vi "get motor settings.vi"(8 "error in (no error)":errorcluster, 10 "motor_settings":T1, 11 "id":i32) -> (0 "error out":errorcluster, 2 "motor_settings out":T1, 3 "function return":i32)   [LabVIEW 2012, in "libximc.lvlib"]
doc: "result_t XIMC_API get_motor_settings (device_t id, motor_settings_t* motor_settings);"
uses:
  libximc.lvlib
  libximc.dll
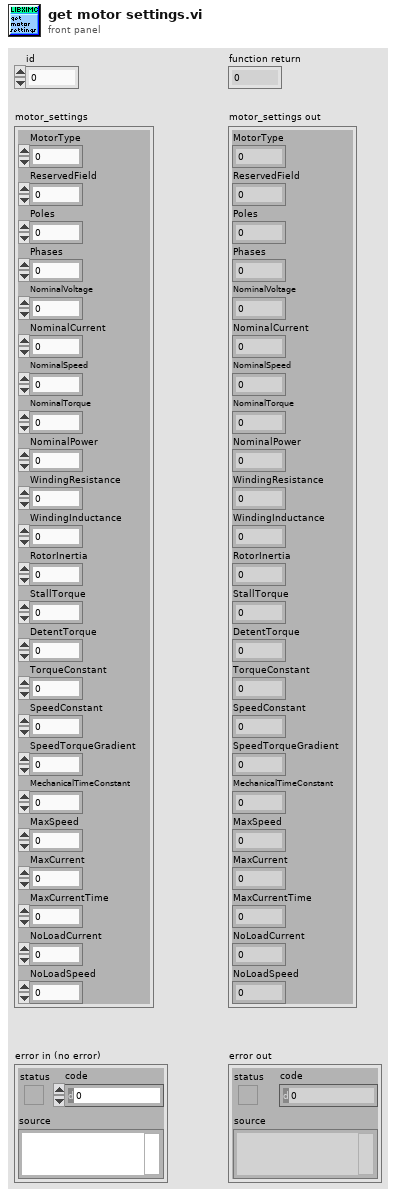
[diagram p1: front panel]
types:
  T1 = cluster{"MotorType":u32, "ReservedField":u32, "Poles":u32, "Phases":u32, "NominalVoltage":sgl, "NominalCurrent":sgl, "NominalSpeed":sgl, "NominalTorque":sgl, "NominalPower":sgl, "WindingResistance":sgl, "WindingInductance":sgl, "RotorInertia":sgl, "StallTorque":sgl, "DetentTorque":sgl, "TorqueConstant":sgl, "SpeedConstant":sgl, "SpeedTorqueGradient":sgl, "MechanicalTimeConstant":sgl, "MaxSpeed":sgl, "MaxCurrent":sgl, "MaxCurrentTime":sgl, "NoLoadCurrent":sgl, "NoLoadSpeed":sgl}
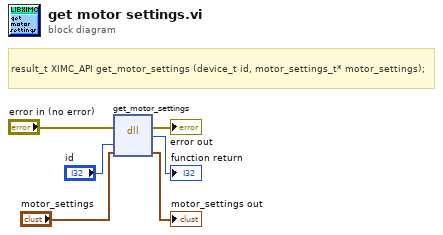
[diagram p0: block diagram]
diagram:
  # "result_t XIMC_API get_motor_settings (device_t id, motor_settings_t* motor_settings);"
  n1 = dll-call lib="E:/labview-2.12.1-Labview_12.0/ximcLVx32/libximc.*" fn="get_motor_settings"(error in="error in (no error)", "id"="id", "motor_settings"="motor_settings") -> (error out=→"error out":errorcluster, →"function return":i32, "motor_settings"=→"motor_settings out":T1)  [unwired: 3 in, 1 out]
